vi "Load Suite from Index.vi"(8 "error in (no error)":errorcluster, 11 "Projext Path":path) -> (0 "error out":errorcluster, 3 "LUnit Test Suite out":refnum<class "LUnit Test Suite.lvclass">)   [LabVIEW 2020, in "Test Finder.lvclass"]
uses:
  Test Finder.lvclass
  LUnit Test Suite.lvclass
  C:/git/astemes-lunit/source/Runnable.lvclass
  Test Finder.lvclass/Test Finder.ctl
  Test Suite Factory/Test Suite Factory.lvclass
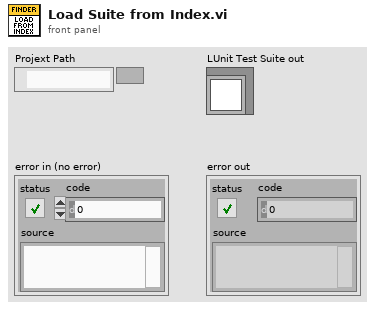
[diagram p1: front panel]
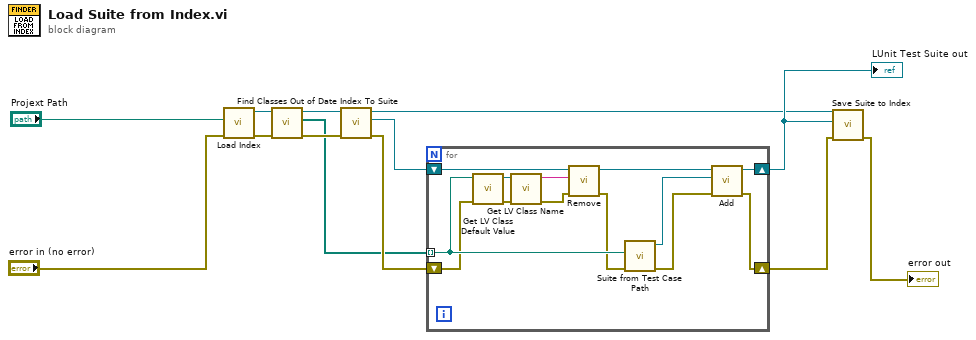
[diagram p0: block diagram]
diagram:
  n1 = call "Load Index.vi"("error in (no error)"="error in (no error)", "Project Path"="Projext Path") -> ("error out"=w3:errorcluster, "Test Finder out"=w2:refnum<class "Test Finder.lvclass">)  [unwired: 8 in]
  n2 = call "Find Classes Out of Date.vi"("error in (no error)"=w3, "Test Finder In"=w2) -> ("error out"=w6:errorcluster, "Outdated Test Class paths"=w4:path[], "Test Finder Out"=w5:refnum<class "Test Finder.lvclass">)  [unwired: 7 in]
  n3 = call "Index To Suite.vi"("error in (no error)"=w6, "Test Finder In"=w5) -> ("error out"=w7:errorcluster, "Suite"=w8:refnum<class "LUnit Test Suite.lvclass">, "Test Finder Out"=w9:refnum<class "Test Finder.lvclass">)  [unwired: 7 in]
  n4 = for {
    tunnel: w4 -> [w18] mode=indexing
    shift-right: [w25] -> w11
    shift-left: w8 -> [w26]
    shift-right: [w24] -> w10
    shift-left: w7 -> [w16]
    n5 = call <vilib>:"Get LV Class Default Value.vi"("error in (no error)"=w16, "class path"=w18) -> ("error out"=w20:errorcluster, "object"=w19:refnum<class>)  [unwired: 8 in]
    n6 = call <vilib>:"Get LV Class Name.vi"("error in (no error)"=w20, "object"=w19) -> ("error out"=w15:errorcluster, "class name"=w17:string)  [unwired: 8 in]
    n7 = call "Remove.vi"("error in (no error)"=w15, "Test to Remove"=w17, "LUnit Test Suite In"=w26) -> ("error out"=w14:errorcluster, "LUnit Test Suite Out"=w21:refnum<class "LUnit Test Suite.lvclass">)  [unwired: 7 in]
    n8 = call "Suite from Test Case Path.vi"("error in (no error)"=w14, "Test Case"=w18) -> ("error out"=w23:errorcluster, "LUnit Test Suite Out"=w22:refnum<class "LUnit Test Suite.lvclass">)  [unwired: 8 in]
    n9 = call "Add.vi"("error in (no error)"=w23, "Runnable"=w22, "LUnit Test Suite In"=w21) -> ("error out"=w24:errorcluster, "LUnit Test Suite Out"=w25:refnum<class "LUnit Test Suite.lvclass">)  [unwired: 7 in]
  }
  "LUnit Test Suite out" <- w11
  n10 = call "Save Suite to Index.vi"("error in (no error)"=w10, "Suite"=w11, "Test Finder In"=w9) -> ("error out"=→"error out":errorcluster)  [unwired: 8 in]
